vi "ROI_calculate_embryo_orientation.vi"(4 "Embryo position 2":cluster{"x(um)":dbl, "y(um)":dbl, "z(um)":dbl}, 7 "Embryo position 1":cluster{"x(um)":dbl, "y(um)":dbl, "z(um)":dbl}) -> (0 "Slope a":dbl, 1 "Embryo's ends":dbl[][](array[numeric]), 2 "b":dbl, 3 "Angle":dbl)   [LabVIEW 2015]
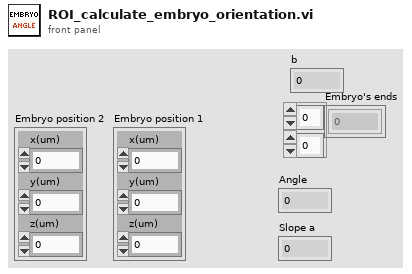
[diagram p1: front panel]
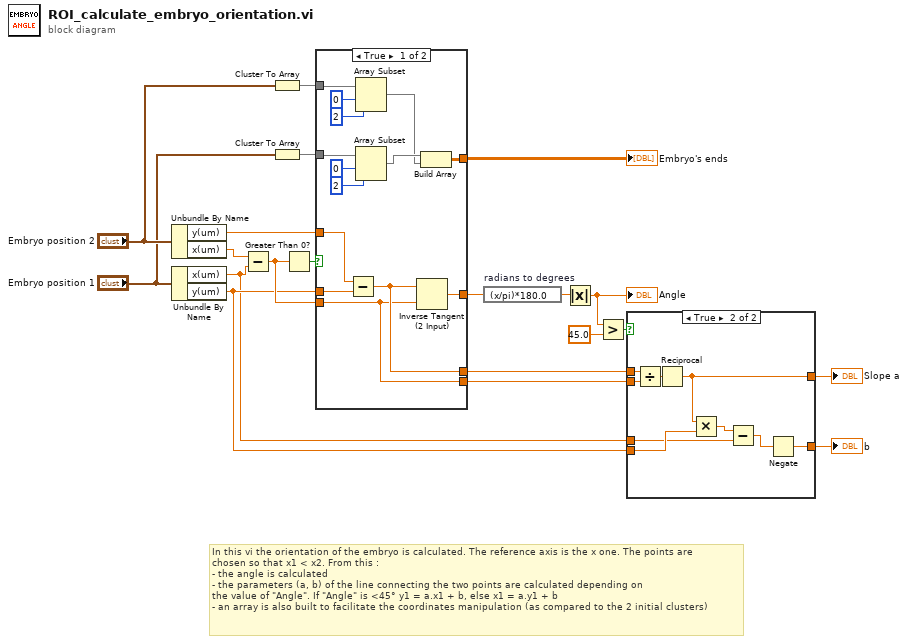
[diagram p0: block diagram]
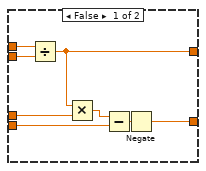
[diagram p2: hidden frame]
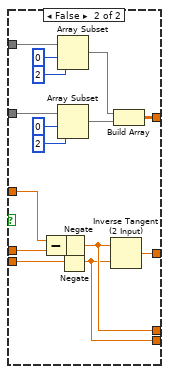
[diagram p3: hidden frame]
diagram:
  # "In this vi the orientation of the embryo is calculated. The reference axis is the x one. The points are\nchosen so that x1 < x2. From this :\n- the angle is calculated\n- the parameters (a, b) of the line connecting the two points are calculated depending on \nthe value of \"Angle\". If \"Angle\" is <45° y1 = a.x1 + b, else x1 = a.y1 + b\n- an array is also built to facilitate the coordinates manipulation (as compared to the 2 initial clusters)"
  n1 = Unbundle By Name("Embryo position 2") -> ("y(um)"=w18:dbl, "x(um)"=w16:dbl)
  n2 = Unbundle By Name("Embryo position 1") -> ("x(um)"=w4:dbl, "y(um)"=w5:dbl)
  n3 = Subtract(x=w16, y=w4) -> (x-y=w19:dbl)
  n4 = Cluster To Array(cluster="Embryo position 2") -> (array=w13:dbl[])
  n5 = Cluster To Array(cluster="Embryo position 1") -> (array=w12:dbl[])
  n6 = Greater Than 0?(x=w19) -> (x > 0?=w20:bool)
  n7 = case shown="True" w20 {
    tunnel: w19 -> [w21 w47]
    tunnel: w18 -> [w33 w49]
    tunnel: w5 -> [w34 w50]
    tunnel: [w32 w46] -> w17
    tunnel: w13 -> [w27 w44]
    tunnel: w12 -> [w26 w38]
    tunnel: [w23 w45] -> w15
    tunnel: [w22 w36] -> w8
    tunnel: [w21 w35] -> w7
    frame True {
      n8 = Subtract(x=w33, y=w34) -> (x-y=w22:dbl)
      n9 = Array Subset(array=w27, index=0, length=2 ("index")) -> (w24:dbl[])
      n10 = Array Subset(array=w26, index=0, length=2 ("index")) -> (w25:dbl[])
      n11 = Inverse Tangent (2 Input)(1:w21, 2:w22) -> (0:w32:dbl)
      n12 = Build Array(w25, w24) -> (w23:dbl[][])
    }
    frame False {
      n13 = Subtract(x=w49, y=w50) -> (x-y=w48:dbl)
      n14 = Array Subset(array=w44, index=0, length=2 ("index")) -> (w41:dbl[])
      n15 = Array Subset(array=w38, index=0, length=2 ("index")) -> (w37:dbl[])
      n16 = Negate(x=w48) -> (-x=w36:dbl)
      n17 = Negate(x=w47) -> (-x=w35:dbl)
      n18 = Inverse Tangent (2 Input)(1:w35, 2:w36) -> (0:w46:dbl)
      n19 = Build Array(w41, w37) -> (w45:dbl[][])
    }
  }
  "Embryo's ends" <- w15
  n20 = expression code="(x/pi)*180.0" "radians to degrees"(w17) -> (w2:dbl)
  n21 = Absolute Value(x=w2) -> (abs(x)=w1:dbl)
  "Angle" <- w1
  n22 = Greater?(x=w1, y=45.0) -> (0:w10:bool)
  n23 = case shown="True" w10 {
    tunnel: w8 -> [w58 w67]
    tunnel: w7 -> [w57 w66]
    tunnel: [w56 w62] -> w6
    tunnel: w5 -> [w53 w61]
    tunnel: w4 -> [w55 w60]
    tunnel: [w51 w59] -> w3
    frame False {
      n24 = Divide(x=w58, y=w57) -> (x/y=w56:dbl)
      n25 = Multiply(x=w56, y=w55) -> (x*y=w54:dbl)
      n26 = Subtract(x=w54, y=w53) -> (x-y=w52:dbl)
      n27 = Negate(x=w52) -> (-x=w51:dbl)
    }
    frame True {
      n28 = Divide(x=w67, y=w66) -> (x/y=w65:dbl)
      n29 = Reciprocal(x=w65) -> (1/x=w62:dbl)
      n30 = Multiply(x=w62, y=w61) -> (x*y=w64:dbl)
      n31 = Subtract(x=w64, y=w60) -> (x-y=w63:dbl)
      n32 = Negate(x=w63) -> (-x=w59:dbl)
    }
  }
  "Slope a" <- w6
  "b" <- w3
